vi "Translation3d_Create_Default.vi"() -> (3 "TRANSLATION3D":T1 {"Z" format="%14.3f"; "Y" format="%14.3f"; "X" format="%14.3f"})   [LabVIEW 2019, in "Trajectory_Library.lvlib"]
doc: "Constructs a Translation3d with X, Y, and Z components equal to zero.\n\nParameters:\n -- None --\n\nReturns\n - TRANSLATION3D - The TRANSLATION3D data structure"
uses:
  Trajectory_Library.lvlib
  TypeDef/TRANSLATION3D.ctl
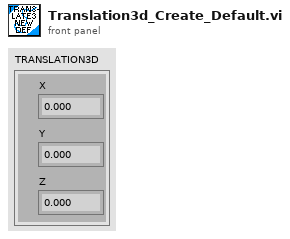
[diagram p1: front panel]
types:
  T1 = typedef "Trajectory_Library.lvlib/TRANSLATION3D.ctl" = cluster{"X":dbl, "Y":dbl, "Z":dbl}
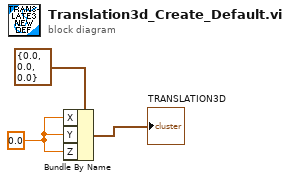
[diagram p0: block diagram]
diagram:
  w2 = 0.0 ("X")
  n1 = Bundle By Name(cluster=T1 {"X"=0.0, "Y"=0.0, "Z"=0.0} ("TRANSLATION"), "X"=w2, "Y"=w2, "Z"=w2) -> (→"TRANSLATION3D":T1)
